vi "Actor Core.vi"(8 "error in":errorcluster, 11 "Main Window in":refnum<class "Main Window.lvclass">) -> (0 "error out":errorcluster, 3 "Actor out":refnum<class "Actor.lvclass">)   [LabVIEW 2021, in "Recipe.lvlib" / "Main Window.lvclass"]
doc: "The user interface for this panel.\n\n----\nPlease see the following web address for additional documentation and tutorial information:\nhttp://www.mooregoodideas.com/mgi-panel-manager/\n\nAuthor: Derek Trepanier\n\nCopyright (c) 2018, Moore Good Ideas, Inc.\n\nAll rights reserved.\n\nRedistribution and use in source and binary forms, with or without modification, are permitted provided that the following conditions are met:\n\n * Redistributions of source code must retain the above copyright notice, this list of conditions and the following disclaimer.\n * Redistributions in binary form must reproduce the above copyright notice, this list of conditions and the following disclaimer in the documentation and/or other materials provided with the distribution.\n * Neither the name of Moore Good Ideas, Inc. nor the names of its contributors may be used to endorse or promote products derived from this software without specific prior written permission.\n\nTHIS SOFTWARE IS PROVIDED BY THE COPYRIGHT HOLDERS AND CONTRIBUTORS \"AS IS\" AND ANY EXPRESS OR IMPLIED WARRANTIES, INCLUDING, BUT NOT LIMITED TO, THE IMPLIED WARRANTIES OF MERCHANTABILITY AND FITNESS FOR A PARTICULAR PURPOSE ARE DISCLAIMED. IN NO EVENT SHALL THE COPYRIGHT OWNER OR CONTRIBUTORS BE LIABLE FOR ANY DIRECT, INDIRECT, INCIDENTAL, SPECIAL, EXEMPLARY, OR CONSEQUENTIAL DAMAGES (INCLUDING, BUT NOT LIMITED TO, PROCUREMENT OF SUBSTITUTE GOODS OR SERVICES; LOSS OF USE, DATA, OR PROFITS; OR BUSINESS INTERRUPTION) HOWEVER CAUSED AND ON ANY THEORY OF LIABILITY, WHETHER IN CONTRACT, STRICT LIABILITY, OR TORT (INCLUDING NEGLIGENCE OR OTHERWISE) ARISING IN ANY WAY OUT OF THE USE OF THIS SOFTWARE, EVEN IF ADVISED OF THE POSSIBILITY OF SUCH DAMAGE."
uses:
  Main Window.lvclass
  C:/Program Files (x86)/National Instruments/LabVIEW 2021/vi.lib/MGI/Panel Manager/Panel Actor/Panel Actor/Panel Actor.lvclass
  <vilib>/ActorFramework/Actor/Actor.lvclass
  <vilib>/ActorFramework/Message Enqueuer/Message Enqueuer.lvclass/Message Enqueuer.ctl
  <vilib>/ActorFramework/Message Enqueuer/Enqueue.vi
  <vilib>/ActorFramework/Stop Msg/Stop Msg.lvclass
  C:/Program Files (x86)/National Instruments/LabVIEW 2021/vi.lib/ActorFramework/Message/Message.lvclass
  <vilib>/ActorFramework/Message Priority Queue/Priority Enqueue.vi
  <vilib>/MGI/Panel Manager/Panel Actor/Panel Actor/Panel Actor.lvclass
  Windows/System32/user32.dll
panel:
  in  "Show Hide Panel":bool
  in  "Header Button":bool
  in  "Window Maximize":bool
  in  "Window Minimize":bool
  in  "Close":bool
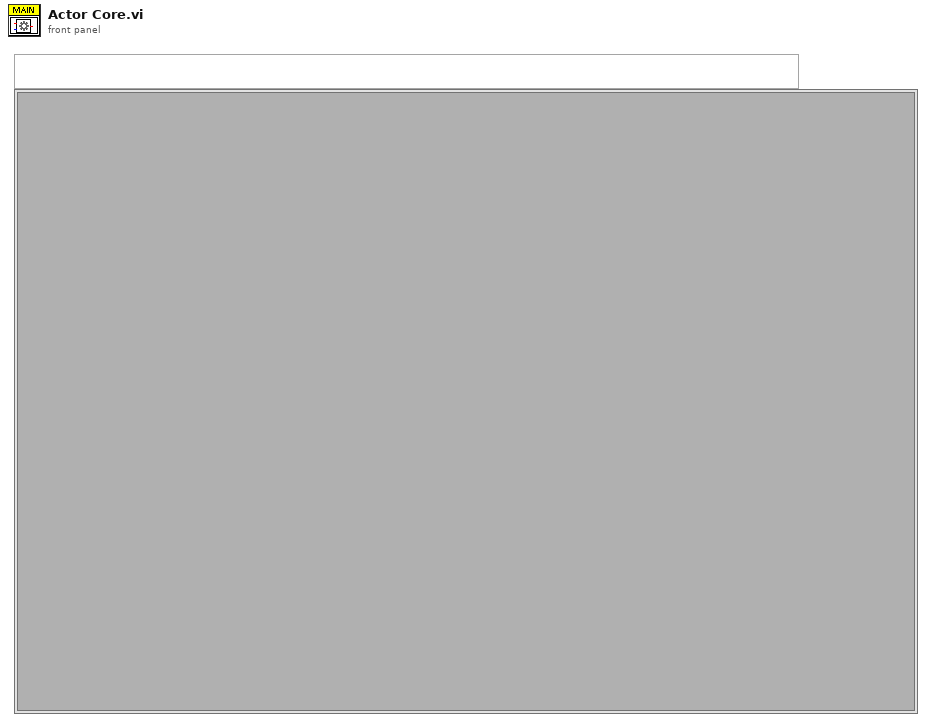
[diagram p1: front panel]
types:
  T1 = enum32{"Invalid", "Standard", "Closed", "Hidden", "Minimized", "Maximized"}
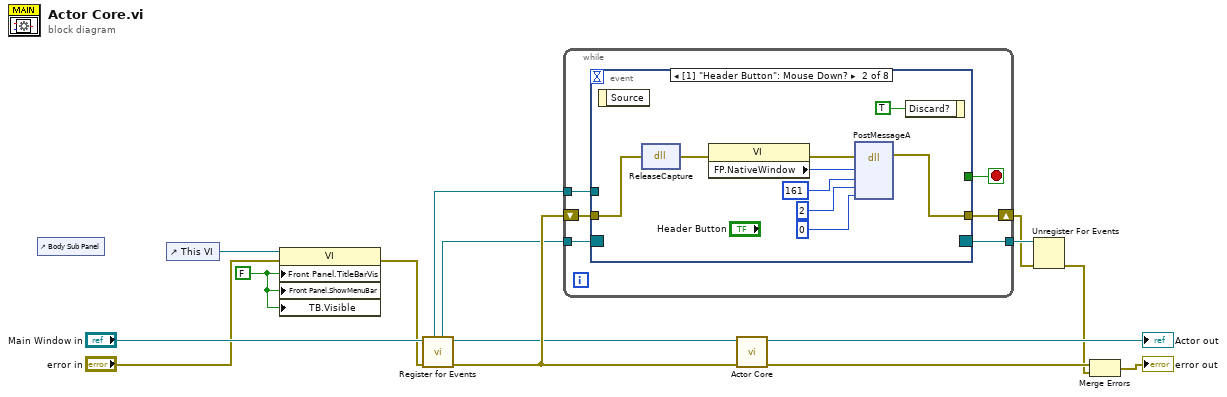
[diagram p0: block diagram]
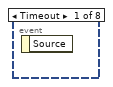
[diagram p2: hidden frame]
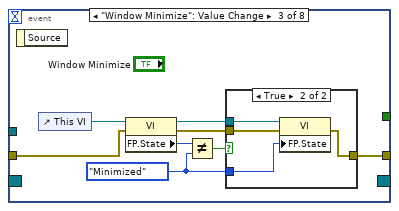
[diagram p3: hidden frame]
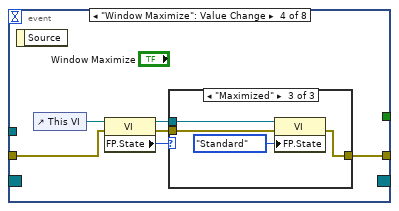
[diagram p5: hidden frame]
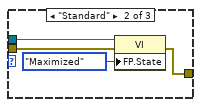
[diagram p7: hidden frame]
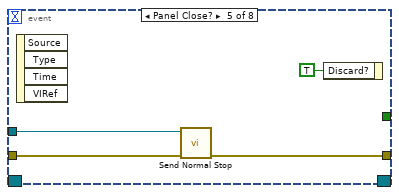
[diagram p8: hidden frame]
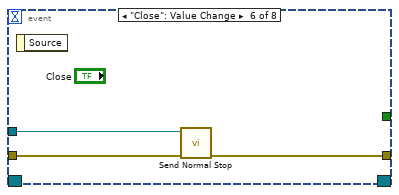
[diagram p9: hidden frame]
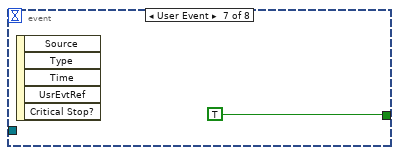
[diagram p10: hidden frame]
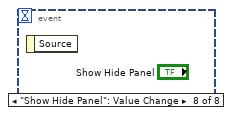
[diagram p11: hidden frame]
diagram:
  w1 = FALSE ("Front Panel Window:Title Bar Visible")
  n1 = control-ref of="Body Sub Panel"() -> ()  [unwired: 1 out]
  n2 = control-ref of="This VI"() -> (w4:refnum<vi>)
  n3 = property class="VI"(reference=w4, error in="error in", "Front Panel.TitleBarVis"=w1, "Front Panel.ShowMenuBar"=w1, "TB.Visible"=w1) -> (error out=w2:errorcluster)  [unwired: 1 out]
  n4 = call <vilib>:"Register for Events.vi"("Error In"=w2, "Panel Actor in"="Main Window in") -> ("Error Out"=w15:errorcluster, "Panel Actor out"=w11:refnum<class "Main Window.lvclass">, "Pnl Actor"=w10:refnum<event-registration>, "Self Enqueuer"=w9:refnum<class "Message Enqueuer.lvclass">)  [unwired: 6 in]
  n5 = while {
    tunnel: w10 -> [w21]
    tunnel: w9 -> [w20]
    shift-right: [w18] -> w6
    shift-left: w15 -> [w17]
    tunnel: [w16] -> w8
    stop <- w19 stop-if-true
    n6 = event shown="[1] \"Header Button\": Mouse Down?" {
      selector: w21 -> [_ _ _ _ _ _ _ _]
      dyn-events: [_ _ _ _ _ _ _ _] -> w16
      timeout: _ -> [_ _ _ _ _ _ _ _]
      tunnel: w20 -> [_ _ _ _ w61 w65 _ _]
      tunnel: [_ _ _ _ _ _ TRUE _] -> w19
      tunnel: [_ w25 w31 w45 w60 w63 _ _] -> w18
      tunnel: w17 -> [_ w29 w32 w48 w59 w64 _ _]
      event Timeout {
        n7 = event-data() -> ()  [unwired: 1 in, 1 out]
      }
      event "Header Button": Mouse Down? {
        n8 = event-data() -> ()  [unwired: 1 in, 1 out]
        n9 = dll-call lib="C:/Windows/System32/user32.dll" fn="ReleaseCapture"(error in=w29) -> (error out=w28:errorcluster)  [unwired: 3 in, 1 out]
        n10 = property class="VI"(error in=w28) -> (error out=w27:errorcluster, "FP.NativeWindow"=w26:u64)  [unwired: 1 in, 1 out]
        n11 = dll-call lib="C:/Windows/System32/user32.dll" fn="PostMessageA"(error in=w27, "arg1"=w26, "arg2"=161, "arg3"=2, "arg4"=0) -> (error out=w25:errorcluster)  [unwired: 7 in, 1 out]
        n12 = event-data("Discard?"=TRUE) -> ()  [unwired: 1 in, 1 out]
      }
      event "Window Minimize": Value Change {
        w34 = T1."Minimized" ("Front Panel Window:State")
        n13 = event-data() -> ()  [unwired: 1 in, 1 out]
        n14 = control-ref of="This VI"() -> (w37:refnum<vi>)
        n15 = property class="VI"(reference=w37, error in=w32) -> (reference out=w38:refnum<vi>, error out=w33:errorcluster, "FP.State"=w36:T1)
        n16 = Not Equal?(x=w36, y=w34) -> (x != y?=w35:bool)
        n17 = case shown="True" w35 {
          tunnel: w38 -> [_ w43]
          tunnel: w34 -> [_ w42]
          tunnel: w33 -> [w39 w41]
          tunnel: [w39 w40] -> w31
          frame False {
          }
          frame True {
            n18 = property class="VI"(reference=w43, error in=w41, "FP.State"=w42) -> (error out=w40:errorcluster)  [unwired: 1 out]
          }
        }
      }
      event "Window Maximize": Value Change {
        n19 = event-data() -> ()  [unwired: 1 in, 1 out]
        n20 = control-ref of="This VI"() -> (w47:refnum<vi>)
        n21 = property class="VI"(reference=w47, error in=w48) -> (reference out=w49:refnum<vi>, error out=w46:errorcluster, "FP.State"=w44:T1)
        n22 = case shown="\"Maximized\"" w44 {
          tunnel: w49 -> [_ w54 w58]
          tunnel: w46 -> [w50 w53 w57]
          tunnel: [w50 w52 w56] -> w45
          frame Default {
          }
          frame "Standard" {
            n23 = property class="VI"(reference=w54, error in=w53, "FP.State"=T1."Maximized" ("Front Panel Window:State")) -> (error out=w52:errorcluster)  [unwired: 1 out]
          }
          frame "Maximized" {
            n24 = property class="VI"(reference=w58, error in=w57, "FP.State"=T1."Standard" ("Front Panel Window:State")) -> (error out=w56:errorcluster)  [unwired: 1 out]
          }
        }
      }
      event Panel Close? {
        n25 = event-data() -> ()  [unwired: 1 in, 4 out]
        n26 = call <vilib>:"Send Normal Stop.vi"("error in (no error)"=w59, "Message Enqueuer"=w61) -> ("error out"=w60:errorcluster)  [unwired: 9 in]
        n27 = event-data("Discard?"=TRUE) -> ()  [unwired: 1 in, 1 out]
      }
      event "Close": Value Change {
        n28 = event-data() -> ()  [unwired: 1 in, 1 out]
        n29 = call <vilib>:"Send Normal Stop.vi"("error in (no error)"=w64, "Message Enqueuer"=w65) -> ("error out"=w63:errorcluster)  [unwired: 9 in]
      }
      event User Event {
        n30 = event-data() -> ()  [unwired: 1 in, 5 out]
      }
      event "Show Hide Panel": Value Change {
        n31 = event-data() -> ()  [unwired: 1 in, 1 out]
      }
    }
  }
  n32 = call-parent "Actor Core.vi"("error in"=w15, "Panel Actor in"=w11) -> ("error out"=w14:errorcluster, "Actor out"=→"Actor out":refnum<class "Actor.lvclass">)  [unwired: 8 in]
  n33 = Unregister For Events(event registration refnum=w8, error in=w6) -> (error out=w5:errorcluster)
  n34 = Merge Errors(w14, w5) -> (→"error out":errorcluster)
